vi "color_alignment.vi"(10 "NXT/EV3":T2, 11 "Begginning color":T1=enum."White") -> (0 "NXT/EV3 2":T2)   [LabVIEW 2016]
uses:
  parametros.ctl
  <vilib>/NXT/Block Support/NXT_InputPort.ctl
  <vilib>/NXT/Subs/LVHSConnector.ctl
  <vilib>/NXT/LegoClasses/BrickReference/BrickReference.lvclass
  <vilib>/NXT/Subs/ColorSensorColors.ctl
  <vilib>/NXT/Block Support/NXT_OutputPort.ctl
  <vilib>/NXT/NXTIO Xnodes/NXTIONodeSubVIs/NXTStopMotors.vi
  <vilib>/NXT/NXTIO Xnodes/NXTIONodeSubVIs/NXTMoveMotors.vi
  <vilib>/NXT/NXTIO Xnodes/AddressXNode/NXTIOAddress.xnode
  <vilib>/NXT/NXTIO Xnodes/NXTIOXNode/NXTIO.xnode
panel:
  out "Collor":T1
  in  "Parâmetros Iniciais":T3={"Gyro Port"=0, "Sensor - Left"=3, "Sensor - Right"=2, "     Color \nSensor Port"=1, "Kp Front"=0.5, "Motor speed"=-15, "Distance to street"=15.0, "Motor speed turns"=16, "Kp Curvas"=0.3} {"Kp Front" format="%.3f"; "Color \nSensor Port" items=["Port 1", "Port 2", "Port 3", "Port 4"]; "Sensor - Right" items=["Port 1", "Port 2", "Port 3", "Port 4"]; "Sensor - Left" items=["Port 1", "Port 2", "Port 3", "Port 4"]; "Gyro Port" items=["Port 1", "Port 2", "Port 3", "Port 4"]}
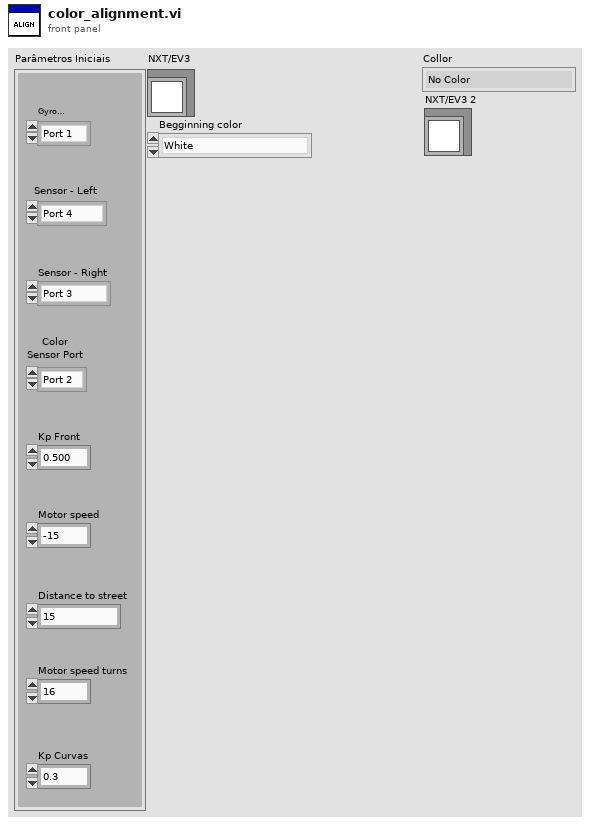
[diagram p1: front panel]
types:
  T1 = typedef "ColorSensorColors.ctl" = enum16{"No Color", "Black", "Blue", "Green", "Yellow", "Red", "White", "Brown"}
  T2 = typedef "LVHSConnector.ctl" = refnum<class "BrickReference.lvclass">
  T3 = typedef "parametros.ctl" = cluster{"Gyro Port":T4, "Sensor - Left":T4, "Sensor - Right":T4, "     Color \nSensor Port":T4, "Kp Front":dbl, "Motor speed":i32, "Distance to street":dbl, "Motor speed turns":i32, "Kp Curvas":dbl}
  T4 = typedef "NXT_InputPort.ctl" = u32
  T5 = typedef "NXT_OutputPort.ctl" = u8
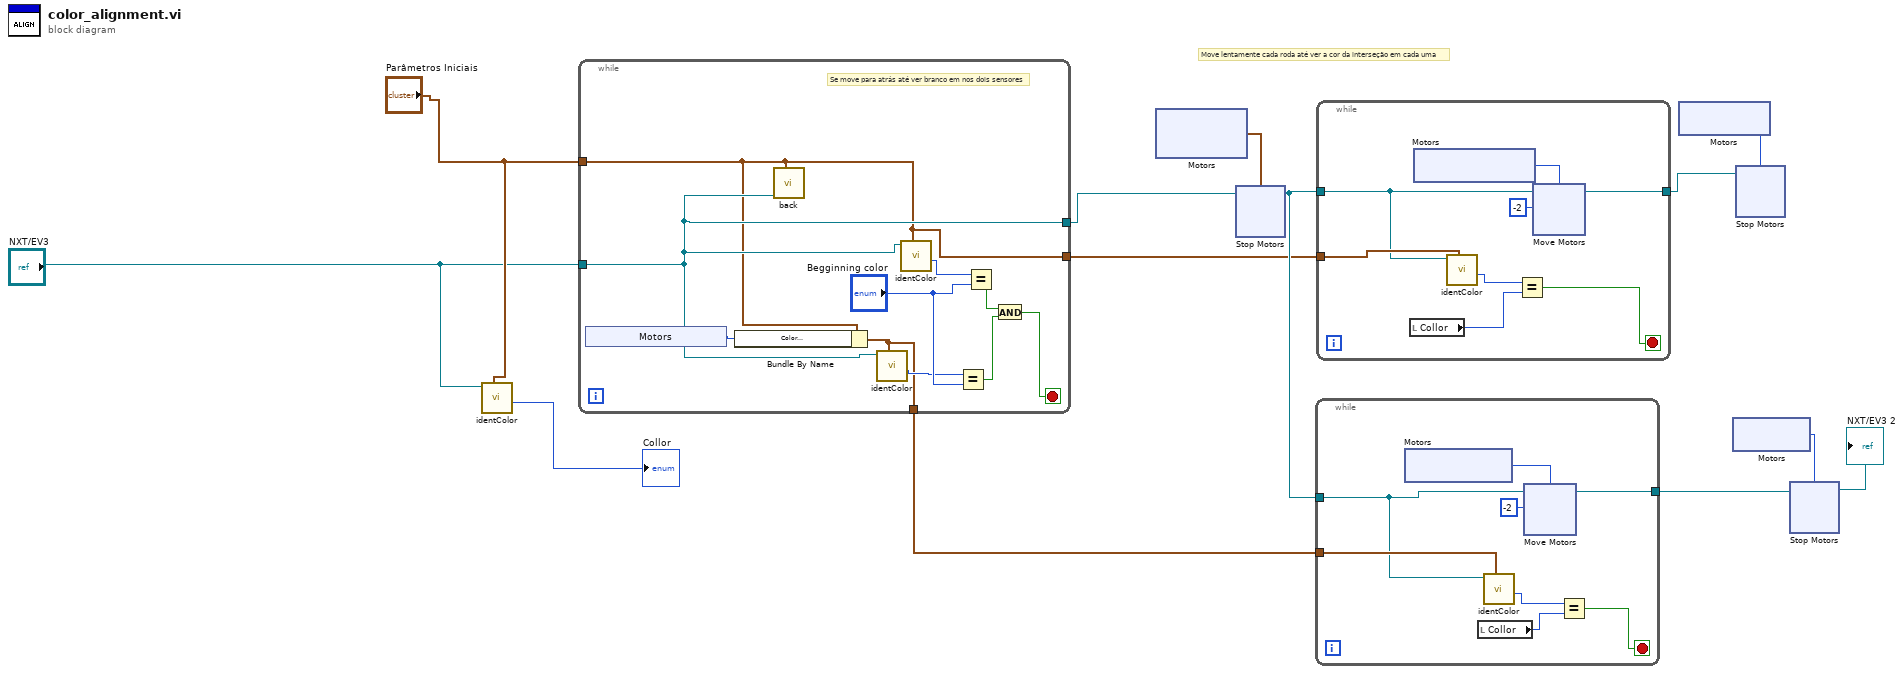
[diagram p0: block diagram]
diagram:
  # "Move lentamente cada roda até ver a cor da interseção em cada uma"
  n1 = call "identColor.vi"("Parâmetros Ini"="Parâmetros Iniciais", "NXT/EV3"="NXT/EV3") -> ("Detected"=→"Collor":T1)  [unwired: 9 in]
  n2 = while {
    tunnel: "NXT/EV3" -> [w18]
    tunnel: "Parâmetros Iniciais" -> [w15]
    tunnel: [w18] -> w10
    tunnel: [w15] -> w2
    tunnel: [w14] -> w1
    stop <- w21 stop-if-true
    # "Se move para atrás até ver branco em nos dois sensores"
    n3 = xnode "Motors"() -> ("Sensor"=w16:T4)
    n4 = Bundle By Name(cluster=w15, "Color \nSensor Port"=w16) -> (w14:T3)
    n5 = call "back.vi"("Parâmetros Ini 2"=w15, "NXT/EV3"=w18) -> ()  [unwired: 9 in, 1 out]
    n6 = call "identColor.vi"("Parâmetros Ini"=w14, "NXT/EV3"=w18) -> ("Detected"=w17:T1)  [unwired: 9 in]
    n7 = call "identColor.vi"("Parâmetros Ini"=w15, "NXT/EV3"=w18) -> ("Detected"=w19:T1)  [unwired: 9 in]
    n8 = Equal?(x=w17, y="Begginning color") -> (x = y?=w22:bool)
    n9 = Equal?(x=w19, y="Begginning color") -> (x = y?=w23:bool)
    n10 = And(x=w23, y=w22) -> (x .and. y?=w21:bool)
  }
  n11 = xnode "Motors"() -> ("Motor"=w11:cluster{"Port":T5, "Port":T5})
  n12 = xnode "Stop Motors"("Motors"=w11, "NXT/EV3"=w10) -> ("NXT/EV3"=w5:T2)
  n13 = while {
    tunnel: w5 -> [w25]
    tunnel: [w28] -> w7
    tunnel: w1 -> [w27]
    stop <- w29 stop-if-true
    n14 = xnode "Motors"() -> ("Motor"=w32:T5)
    n15 = local read "Collor"() -> (w30:T1)
    n16 = call "identColor.vi"("Parâmetros Ini"=w27, "NXT/EV3"=w25) -> ("Detected"=w26:T1)  [unwired: 9 in]
    n17 = xnode "Move Motors"("Power/Speed 1"=i8 -2, "Motors"=w32, "NXT/EV3"=w25) -> ("NXT/EV3"=w28:T2)
    n18 = Equal?(x=w26, y=w30) -> (x = y?=w29:bool)
  }
  n19 = while {
    tunnel: w5 -> [w42]
    tunnel: [w46] -> w6
    tunnel: w2 -> [w43]
    stop <- w44 stop-if-true
    n20 = local read "Collor"() -> (w45:T1)
    n21 = xnode "Motors"() -> ("Motor"=w48:T5)
    n22 = call "identColor.vi"("Parâmetros Ini"=w43, "NXT/EV3"=w42) -> ("Detected"=w41:T1)  [unwired: 9 in]
    n23 = Equal?(x=w41, y=w45) -> (x = y?=w44:bool)
    n24 = xnode "Move Motors"("Power/Speed 1"=i8 -2, "Motors"=w48, "NXT/EV3"=w42) -> ("NXT/EV3"=w46:T2)
  }
  n25 = xnode "Motors"() -> ("Motor"=w9:T5)
  n26 = xnode "Motors"() -> ("Motor"=w8:T5)
  n27 = xnode "Stop Motors"("Motors"=w9, "NXT/EV3"=w6) -> ()  [unwired: 1 out]
  n28 = xnode "Stop Motors"("Motors"=w8, "NXT/EV3"=w7) -> ("NXT/EV3"=→"NXT/EV3 2":T2)
